vi "Detector Init.vi"(8 "error in (no error)":errorcluster, 10 "Detector Config":T1={"Detector"=0, "Offsets"=[[0, 0, 0, 0, 0, 0, 0, 0, 0, 0, 0, 0, 0, 0, 0, 0, 0, 0, 0, 0, 0, 0, 0, 0, 0, 0, 0, 0, 0, 0, 0, 0]], "Detector Computer"={"Machine"="192.168.121.11", "Password"="", "FITS File Path"="", "Port"=44444, "Header Path"="", "Name"=""}, "FITS hdr template0"=path "", "FITS hdr template1"=path "", "FITS Data File Path"=path "", "FITS Detector Settings"={"Exp Time Short"=0.0, "# of Frames"=0.0, "Exp Time Long"=0.0, "# of Groups"=0.0, "Object Name"="", "Object"="", "Obs Type"="", "Image Type"="", "Observer"="", "Observer Affiliation"=""}, "Sim Folder"=path "", "Integration Mode"=enum."SSR", "Integration Time"=0.0, "Frame Int Time"=0.0} {"Offsets" format="%04x"; "Detector" items=["0", "1", "2"]}, 11 "RIMAS Detector in":refnum<class "RIMAS Detector.lvclass">) -> (0 "error out":errorcluster, 2 "Log Messages":string[](array[string]), 3 "RIMAS Detector out":refnum<class "RIMAS Detector.lvclass">)   [LabVIEW 2024, in "RIMAS Detector.lvclass"]
uses:
  RIMAS Detector.lvclass
  RIMAS Detector Config.ctl
  RIMAS Detector Server Config.ctl
  RIMAS Observation Config.ctl
  Detector enum Detector Integration Mode.ctl
  RIMAS Detector.lvclass/RIMAS Detector.ctl
  Detector Class.lvclass
panel:
  # "sec"
  # "sec"
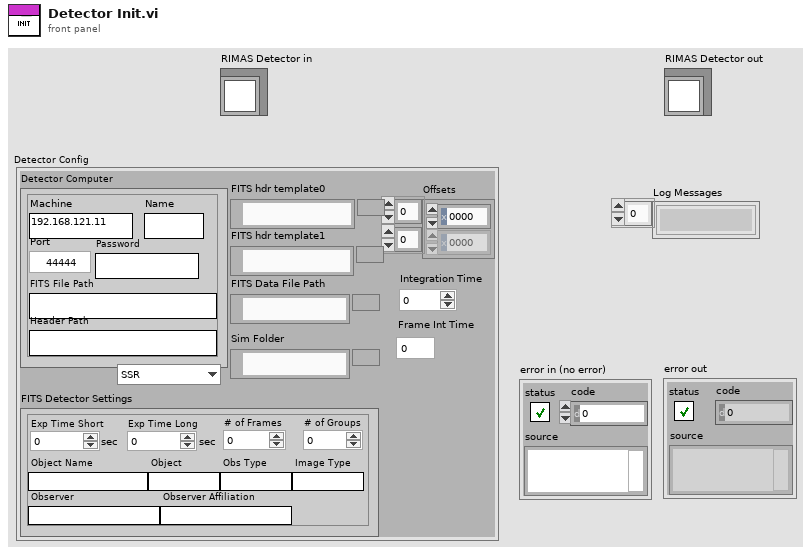
[diagram p1: front panel]
types:
  T1 = typedef "RIMAS Detector Config.ctl" = cluster{"Detector":u16, "Offsets":u16[][], "Detector Computer":T2, "FITS hdr template0":path, "FITS hdr template1":path, "FITS Data File Path":path, "FITS Detector Settings":T3, "Sim Folder":path, "Integration Mode":T4, "Integration Time":dbl, "Frame Int Time":dbl}
  T2 = typedef "RIMAS Detector Server Config.ctl" = cluster{"Machine":string, "Password":string, "FITS File Path":string, "Port":u16, "Header Path":string, "Name":string}
  T3 = typedef "RIMAS Observation Config.ctl" = cluster{"Exp Time Short":dbl, "# of Frames":dbl, "Exp Time Long":dbl, "# of Groups":dbl, "Object Name":string, "Object":string, "Obs Type":string, "Image Type":string, "Observer":string, "Observer Affiliation":string}
  T4 = typedef "Detector enum Detector Integration Mode.ctl" = enum16{"SSR", "CDS", "MEAN", "MEDIAN", "MODE", "MIIN", "MAX"}
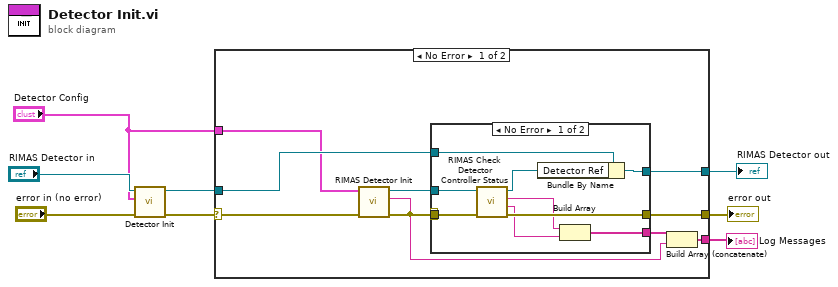
[diagram p0: block diagram]
diagram:
  n1 = call-parent "Detector Init.vi"("error in (no error)"="error in (no error)", "Detector Config"="Detector Config", "Detector Class in"="RIMAS Detector in") -> ("error out"=w6:errorcluster, "Detector Class out"=w5:refnum<class "RIMAS Detector.lvclass">)  [unwired: 6 in, 1 out]
  n2 = case shown="No Error" w6 {
    selector: w6 -> [w9 w31]
    tunnel: w5 -> [w17 w30]
    tunnel: [w16 w30] -> w4
    tunnel: [w15 w31] -> w3
    tunnel: [w11 _] -> w2
    tunnel: "Detector Config" -> [w10 _]
    frame No Error {
      n3 = call "RIMAS Detector Init.vi"("Error In"=w9, "Detector Config"=w10) -> ("Error Out"=w14:errorcluster, "Log Message"=w12:string, "Detector Ref"=w18:refnum<k5>)  [unwired: 7 in]
      n4 = case shown="No Error" w14 {
        selector: w14 -> [w22 w28]
        tunnel: w18 -> [w27 _]
        tunnel: w14 -> [_ _]
        tunnel: w17 -> [w26 w29]
        tunnel: [w24 w29] -> w16
        tunnel: [w23 w28] -> w15
        tunnel: [w19 _] -> w13
        frame No Error {
          n5 = call "RIMAS Check Detector Controller Status.vi"("error in (no error)"=w22, "Detector Ref  in"=w27) -> ("error out"=w23:errorcluster, "Status Controllers"=w20:string, "Status Headers"=w21:string, "Detector Ref out"=w25:refnum<k5>)  [unwired: 6 in]
          n6 = Bundle By Name(cluster=w26, "Detector Ref"=w25) -> (w24:refnum<class "RIMAS Detector.lvclass">)
          n7 = Build Array(w21, w20) -> (w19:string[])
        }
        frame Error {
        }
      }
      n8 = Build Array (concatenate)(w13, w12) -> (w11:string[])
    }
    frame Error {
    }
  }
  "error out" <- w3
  "RIMAS Detector out" <- w4
  "Log Messages" <- w2
